vi "Assert Reuse Component.vi"(4 "Execution time (s)":dbl=-1.0, 5 "Assert Only? (F)":bool, 6 "error code (1)":i32=1, 7 "Label":string, 8 "error in (no error)":errorcluster, 11 "ACME Value":dbl) -> (0 "error out":errorcluster)   [LabVIEW 2020, in "Assert.ACME.lvclass"]
uses:
  Assert.ACME.lvclass
  classes/Assert/Assert.lvclass
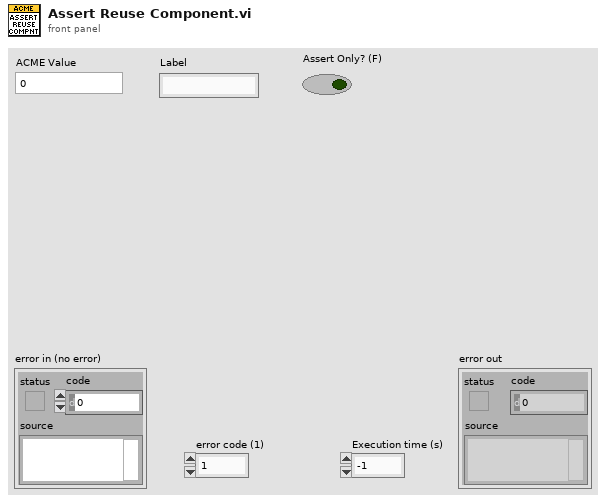
[diagram p1: front panel]
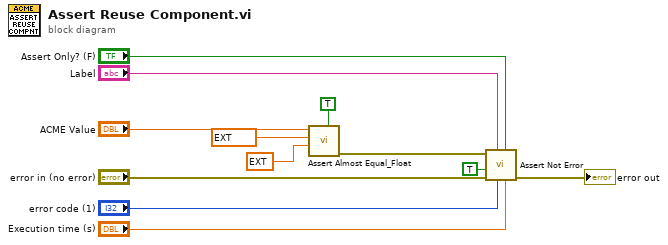
[diagram p0: block diagram]
diagram:
  n1 = call "Assert Almost Equal_Float.vi"("Assert Only? (F)"=TRUE, "Tolerance"=ext 0.01 ("Y"), "Y"=ext 3.14159, "X"="ACME Value") -> ("error out"=w4:errorcluster)  [unwired: 6 in, 1 out]
  n2 = call "Assert Not Error.vi"("Execution time (s)"="Execution time (s)", "Assert Only? (F)"="Assert Only? (F)", "error code (1)"="error code (1)", "Label"="Label", "error in (no error)"="error in (no error)", "Register with caller test (F)"=TRUE, "Not Error?"=w4) -> ("error out"=→"error out":errorcluster)  [unwired: 3 in, 1 out]
